vi "saturate-detect.vi"(6 "bound":sgl, 11 "x":sgl) -> (0 "saturated":bool, 2 "sat(x)":sgl)   [LabVIEW 2015]
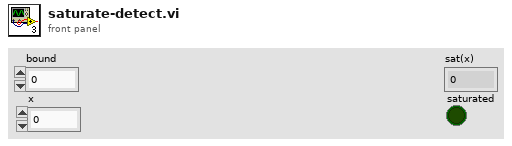
[diagram p1: front panel]
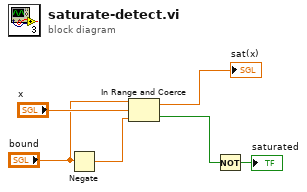
[diagram p0: block diagram]
diagram:
  n1 = Negate(x="bound") -> (-x=w4:sgl)
  n2 = In Range and Coerce(upper limit="bound", x="x", lower limit=w4) -> (coerced(x)=→"sat(x)":sgl, In Range?=w1:bool)
  n3 = Not(x=w1) -> (.not. x?=→"saturated":bool)
